vi "_mzData Description.vi"(1 "Sample Name":string) -> (0 "Output XML":string)   [LabVIEW 2012]
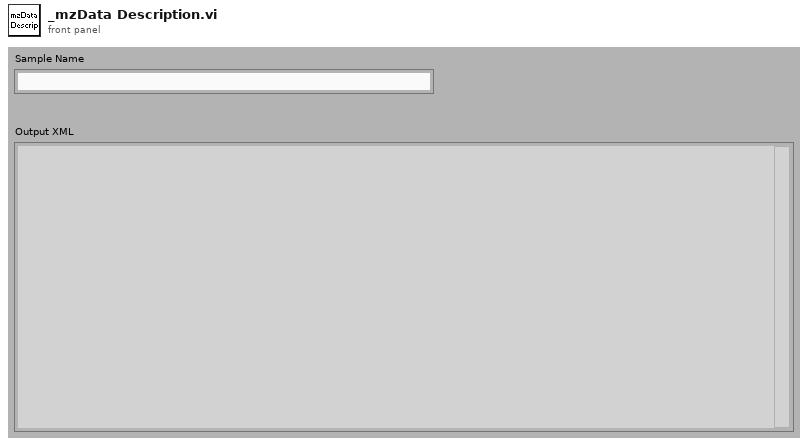
[diagram p1: front panel]
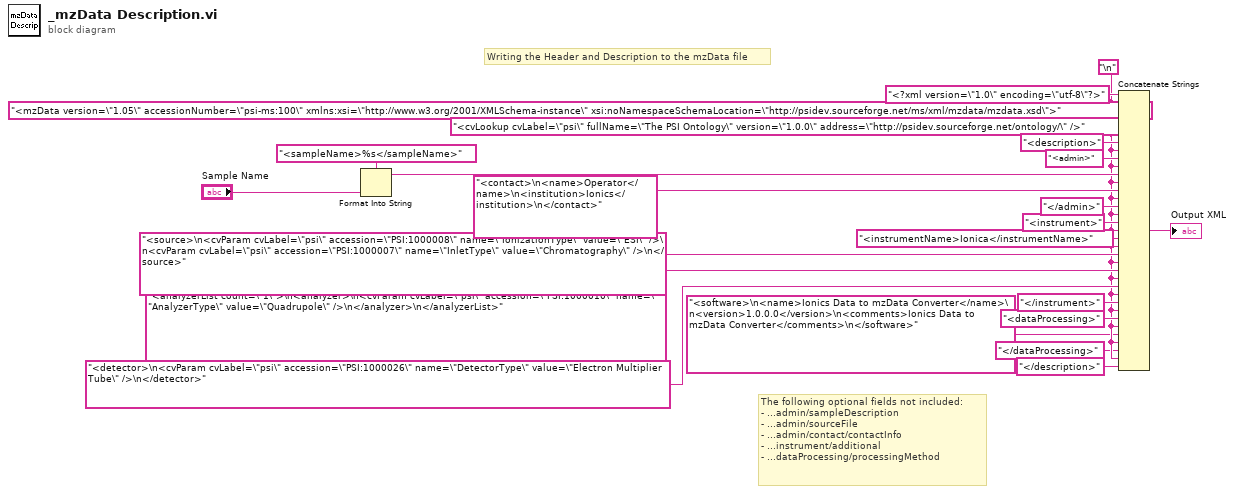
[diagram p0: block diagram]
diagram:
  w5 = "\n"
  # "Writing the Header and Description to the mzData file"
  # "The following optional fields not included:\n- ...admin/sampleDescription\n- ...admin/sourceFile\n- ...admin/contact/contactInfo\n- ...instrument/additional\n- ...dataProcessing/processingMethod"
  n1 = Format Into String(format string="<sampleName>%s</sampleName>", "Sample Name") -> (resulting string=w15:string)  [unwired: 2 in, 1 out]
  n2 = Concatenate Strings("<?xml version=\"1.0\" encoding=\"utf-8\"?>", w5, "<mzData version=\"1.05\" accessionNumber=\"psi-ms:100\" xmlns:xsi=\"http://www.w3.org/2001/XMLSchema-instance\" xsi:noNamespaceSchemaLocation=\"http://psidev.sourceforge.net/ms/xml/mzdata/mzdata.xsd\">", w5, "<cvLookup cvLabel=\"psi\" fullName=\"The PSI Ontology\" version=\"1.0.0\" address=\"http://psidev.sourceforge.net/ontology/\" />", w5, "<description>", w5, "<admin>", w5, w15, w5, "<contact>\n<name>Operator</name>\n<institution>Ionics</institution>\n</contact>", w5, "</admin>", w5, "<instrument>", w5, "<instrumentName>Ionica</instrumentName>", w5, "<source>\n<cvParam cvLabel=\"psi\" accession=\"PSI:1000008\" name=\"IonizationType\" value=\"ESI\" />\n<cvParam cvLabel=\"psi\" accession=\"PSI:1000007\" name=\"InletType\" value=\"Chromatography\" />\n</source>", w5, "<analyzerList count=\"1\">\n<analyzer>\n<cvParam cvLabel=\"psi\" accession=\"PSI:1000010\" name=\"AnalyzerType\" value=\"Quadrupole\" />\n</analyzer>\n</analyzerList>", w5, "<detector>\n<cvParam cvLabel=\"psi\" accession=\"PSI:1000026\" name=\"DetectorType\" value=\"Electron Multiplier Tube\" />\n</detector>", w5, "</instrument>", w5, "<dataProcessing>", w5, "<software>\n<name>Ionics Data to mzData Converter</name>\n<version>1.0.0.0</version>\n<comments>Ionics Data to mzData Converter</comments>\n</software>", w5, "</dataProcessing>", w5, "</description>") -> (→"Output XML":string)
